vi "Read Waveform Measurement (Histogram).vi"(0 "VISA resource name":refnum<visa-resource-name>, 1 "Maximum Time (25000ms)":u32=25000, 7 "Function (0:Wfm Ct)":u16(ring) items=["Wfm Ct", "Median", "Pk-Pk", "Hits in Box", "Max", "Mean", "Peak Hits", "Min", "St Dev", "Sigma1", "Sigma2", "Sigma3"], 11 "error in (no error)":errorcluster) -> (4 "VISA resource name out":refnum<visa-resource-name>, 6 "Measurement":dbl, 15 "error out":errorcluster)   [LabVIEW 2011, in "Tektronix 7000 Series.lvlib"]
doc: "Initiates an acquisition on the channels that you enable with the Configure Channel VI. This VI then waits for the acquisition to complete, obtains a waveform measurement on the channel you specify, and returns the measurement value.\n\n<B>Note:</B> You must configure the histogram before you run this VI."
uses:
  Tektronix 7000 Series.lvlib
  Low Level/Fetch Waveform Measurement (Histogram).vi
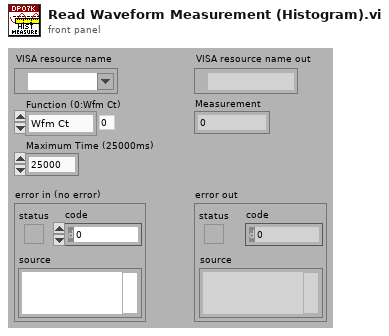
[diagram p1: front panel]
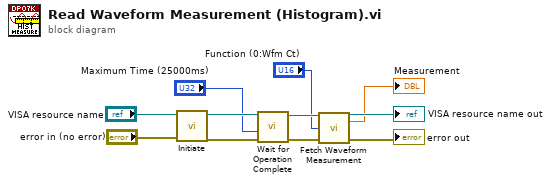
[diagram p0: block diagram]
diagram:
  n1 = call "Initiate.vi"("error in (no error)"="error in (no error)", "VISA resource name"="VISA resource name") -> ("error out"=w9:errorcluster, "VISA resource name out"=w8:refnum<visa-resource-name>)  [unwired: 8 in]
  n2 = call "Wait for Operation Complete.vi"("error in (no error)"=w9, "Maximum Time (2000ms)"="Maximum Time (25000ms)", "VISA resource name"=w8) -> ("error out"=w5:errorcluster, "VISA resource name out"=w6:refnum<visa-resource-name>)  [unwired: 7 in]
  n3 = call-poly "Fetch Waveform Measurement.vi"("VISA resource name"=w6, "Function (0:Wfm Ct)"="Function (0:Wfm Ct)", "error in (no error)"=w5) -> ("VISA resource name out"=→"VISA resource name out":refnum<visa-resource-name>, "Measurement"=→"Measurement":dbl, "error out"=→"error out":errorcluster)  [unwired: 10 in]
